vi "Set Process Model.vi"(8 "error in (no error)":errorcluster, 10 "Process Model":refnum<class "SequenceFile.lvclass">, 11 "Execution in":refnum<class "Execution.lvclass">) -> (0 "error out":errorcluster, 3 "Execution out":refnum<class "Execution.lvclass">)   [LabVIEW 2020, in "TSnax.lvlib" / "Execution.lvclass"]
uses:
  Execution.lvclass
  Execution.lvclass/Execution.ctl
  SequenceFile/SequenceFile.lvclass
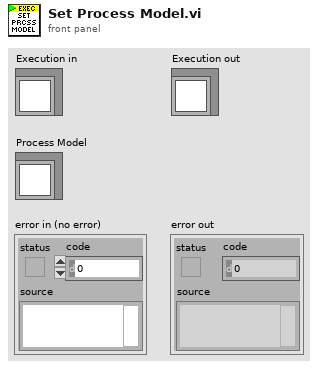
[diagram p1: front panel]
types:
  T1 = typedef "TSnax.lvlib/SequenceFile.lvclass/SequenceFile Type.ctl" = enum16{"Normal", "Model", "Front End Callbacks", "Station Callbacks", "Template"}
  T2 = typedef "TSnax.lvlib/Execution.lvclass/Ref Data.ctl" = cluster{"Parameters":refnum<class "PropertyObject.lvclass">, "Client Sequence":refnum<class "SequenceFile.lvclass">, "Process Model":refnum<class "SequenceFile.lvclass">, "Entry Sequence":string, "Execution":refnum<k7>, "Report":refnum<class "Report.lvclass">, "Options":T3}
  T3 = typedef "TSnax.lvlib/Execution.lvclass/Execution Options.ctl" = cluster{"Use Default Model":bool, "Release Related Sessions":bool}
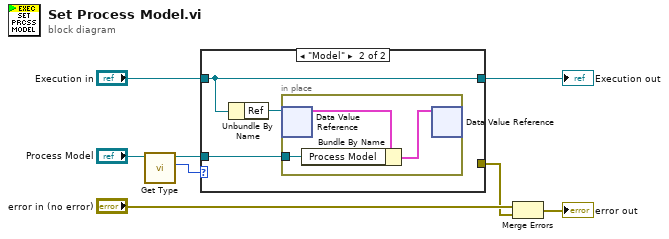
[diagram p0: block diagram]
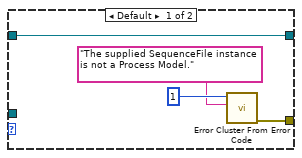
[diagram p2: hidden frame]
diagram:
  n1 = call "Get Type.vi"("SequenceFile in"="Process Model") -> ("Type"=w5:T1, "SequenceFile out"=w4:refnum<class "SequenceFile.lvclass">)  [unwired: 8 in, 1 out]
  n2 = case shown="\"Model\"" w5 {
    tunnel: "Execution in" -> [w12 w14]
    tunnel: w4 -> [_ w13]
    tunnel: [w12 w14] -> w3
    tunnel: [w9 _] -> w1
    frame Default {
      n3 = call <vilib>:"Error Cluster From Error Code.vi"("error message (\"\")"="The supplied SequenceFile instance is not a Process Model." ("error message (\"\")"), "error code (0)"=1) -> ("error out"=w9:errorcluster)  [unwired: 7 in]
    }
    frame "Model" {
      n4 = Unbundle By Name(w14) -> ("Ref"=w15:refnum<data-value>)
      n5 = in-place {
        in-place-border: w13 -> [w16]
        n6 = in-place-dvr #1(w15) -> (w18:T2)  [unwired: 1 out]
        n7 = Bundle By Name(cluster=w18, "Process Model"=w16) -> (w17:T2)
        n8 = in-place-dvr #1(w17) -> ()  [unwired: 2 out]
      }
    }
  }
  "Execution out" <- w3
  n9 = Merge Errors("error in (no error)", w1) -> (→"error out":errorcluster)
